vi "Find Top Caller.vi"(4 "error in":errorcluster, 5 "Level in":i32, 7 "VI Ref":refnum<vi>) -> (0 "error out":errorcluster, 1 "Highest Level":i32, 2 "Highest VI Ref":refnum<vi>, 3 "dup VI Ref":refnum<vi>)   [LabVIEW 2025, in "XNode Support.lvlib"]
doc: "Finds the highest level caller of the VI"
uses:
  XNode Support.lvlib
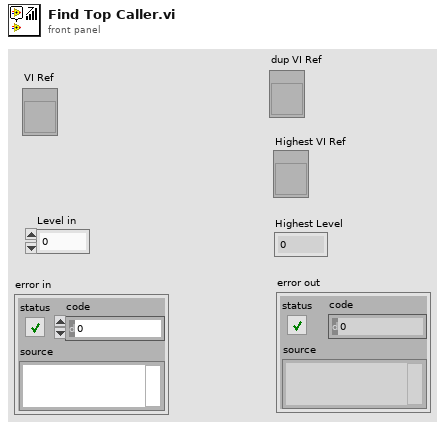
[diagram p1: front panel]
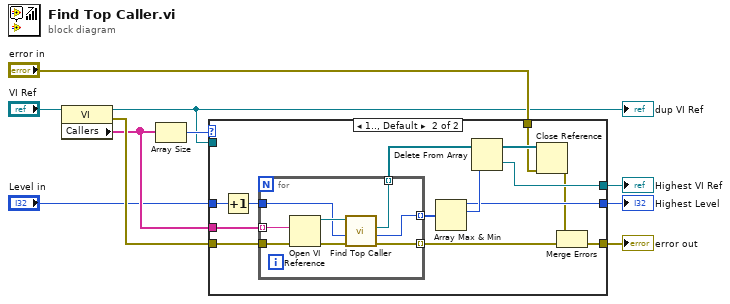
[diagram p0: block diagram]
diagram:
  n1 = property class="VI"(reference="VI Ref") -> (reference out=w4:refnum<vi>, error out=w9:errorcluster, "Callers"=w6:string[])  [unwired: 1 in]
  "dup VI Ref" <- w4
  n2 = Array Size(array=w6) -> (size(s)=w5:i32)
  n3 = case shown="1.., Default" w5 {
    tunnel: w9 -> [w11 w27]
    tunnel: "error in" -> [_ w17]
    tunnel: [w11 w25] -> w7
    tunnel: w6 -> [_ w24]
    tunnel: w4 -> [w13 _]
    tunnel: [w13 w19] -> w3
    tunnel: [w12 w20] -> w2
    tunnel: "Level in" -> [w12 w15]
    frame 0 {
    }
    frame 1.., Default {
      n4 = Increment(x=w15) -> (x+1=w16:i32)
      n5 = for {
        tunnel: w24 -> [w35] mode=indexing
        tunnel: w16 -> [w30]
        tunnel: w27 -> [w33]
        tunnel: [w31] -> w22 mode=indexing
        tunnel: [w28] -> w26 mode=indexing
        tunnel: [w29] -> w23 mode=indexing
        n6 = Open VI Reference(vi path=w35, error in (no error)=w33) -> (vi reference=w34:refnum<vi>, error out=w32:errorcluster)  [unwired: 4 in]
        n7 = call "Find Top Caller.vi"("error in"=w32, "Level in"=w30, "VI Ref"=w34) -> ("error out"=w28:errorcluster, "Highest Level"=w29:i32, "Highest VI Ref"=w31:refnum<vi>)  [unwired: 1 in, 1 out]
      }
      n8 = Array Max & Min(array=w23) -> (max value=w20:i32, max index (indices)=w21:i32)  [unwired: 2 out]
      n9 = Delete From Array(array=w22, index=w21) -> (deleted portion=w19:refnum<vi>, array with subset deleted=w18:refnum<vi>[])  [unwired: 1 in]
      n10 = Close Reference(reference=w18, error in (no error)=w17) -> (error out=w14:errorcluster)
      n11 = Merge Errors(w14, w26) -> (w25:errorcluster)
    }
  }
  "error out" <- w7
  "Highest VI Ref" <- w3
  "Highest Level" <- w2
